vi "Simple Client - Front Panel.vi"() -> ()   [LabVIEW 2011]
panel:
  in  "Exit":bool
  out "Value over Time":dbl(graph)
  out "Value":dbl(knob) scale=0.0..10.0
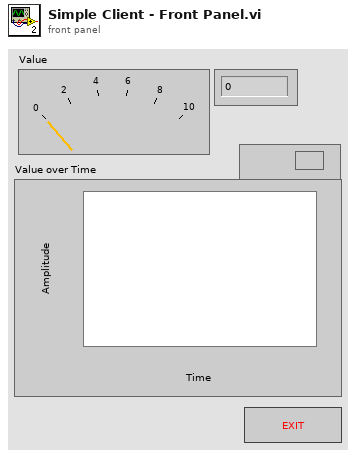
[diagram p1: front panel]
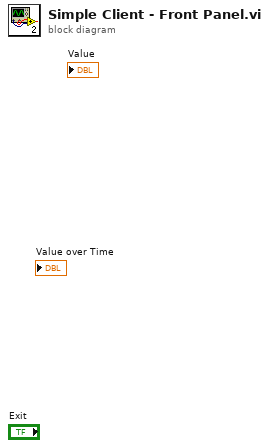
[diagram p0: block diagram]
diagram:
